vi "send status update.vi"(6 "status (F)":bool, 9 "subject":string="comms loop", 11 "RT Queues":T1) -> (3 "RT Queues out":T1)   [LabVIEW 2018]
uses:
  Type Defs/Queues cluster.ctl
  ICL-LabVIEW_General/Message Scheduler/message scheduler.lvclass
  Queue VIs/En-queue RT message element.vi
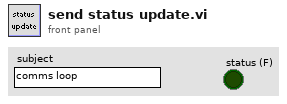
[diagram p1: front panel]
types:
  T1 = typedef "Queues cluster.ctl" = cluster{"RT Message":refnum<queue>, "RT Comms":refnum<queue>, "RT Data":refnum<queue>, "RT FIFO":refnum<queue>, "message scheduler":refnum<class "message scheduler.lvclass">}
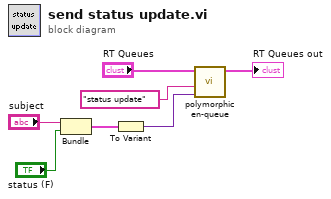
[diagram p0: block diagram]
diagram:
  n1 = Bundle("subject"="subject", "status (F)"="status (F)") -> (w3:cluster{"subject":string, "status (F)":bool})  [unwired: 1 in]
  n2 = To Variant(anything=w3) -> (Variant=w7:variant)
  n3 = call-poly "polymorphic en-queue.vi"("Data"=w7, "Message"="status update", "RT Queues"="RT Queues") -> ("RT Queues out"=→"RT Queues out":T1)  [unwired: 8 in]
